vi "室外火焰对话框.vi"   [LabVIEW 2018]
types:
  T1 = enum32{"Invalid", "Standard", "Closed", "Hidden", "Minimized", "Maximized"}
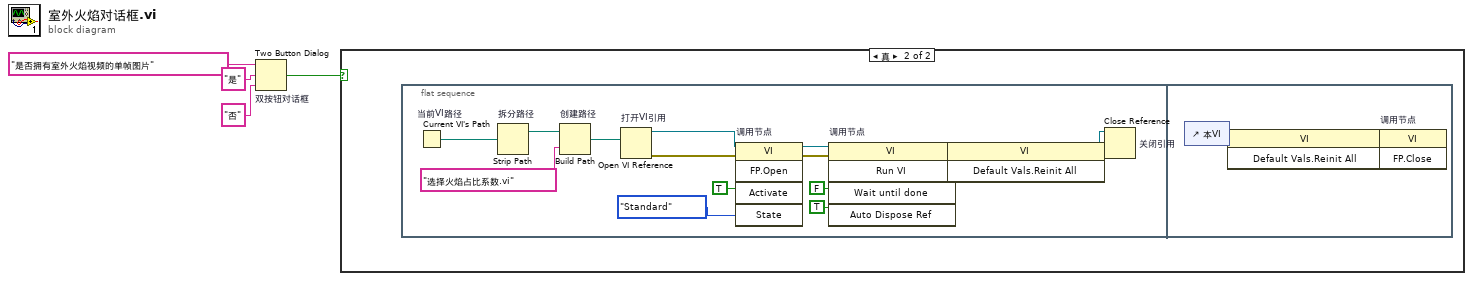
[diagram p0: block diagram]
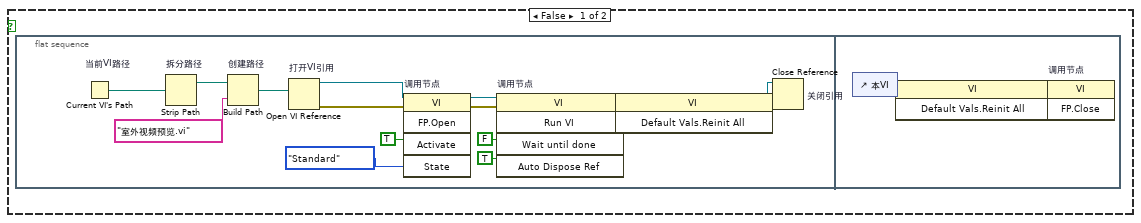
[diagram p2: hidden frame]
diagram:
  n1 = Two Button Dialog "双按钮对话框"(message="是否拥有室外火焰视频的单帧图片" ("消息"), 1:"否" ("F按钮名称（“取消”）"), 2:"是" ("T按钮名称（“确定”）")) -> (T button?=w1:bool)
  n2 = case shown="真" w1 {
    frame False {
      n3 = flat-sequence {
        frame #0 {
          n4 = Current VI's Path "当前VI路径"() -> (path=w16:path)
          n5 = Strip Path "拆分路径"(path=w16) -> (stripped path=w20:path)  [unwired: 1 out]
          n6 = Build Path "创建路径"(base path=w20, name or relative path="室外视频预览.vi" ("名称或相对路径")) -> (appended path=w17:path)
          n7 = Open VI Reference "打开VI引用"(vi path=w17) -> (vi reference=w14:refnum<vi>, error out=w13:errorcluster)  [unwired: 5 in]
          n8 = invoke on="调用节点" class="VI" method="FP.Open"(reference=w14, error in=w13, "Activate"=TRUE ("激活？"), "State"=T1."Standard" ("状态")) -> (reference out=w12:refnum<vi>, error out=w11:errorcluster)  [unwired: 1 in, 3 out]
          n9 = invoke on="调用节点" class="VI" method="Run VI"(reference=w12, error in=w11, "Wait until done"=FALSE ("结束前等待"), "Auto Dispose Ref"=TRUE ("自动销毁引用")) -> (reference out=w8:refnum<vi>, error out=w5:errorcluster)  [unwired: 1 in, 3 out]
          n10 = invoke class="VI" method="Default Vals.Reinit All"(reference=w8, error in=w5) -> (reference out=w7:refnum<vi>, error out=w6:errorcluster)  [unwired: 1 in, 1 out]
          n11 = Close Reference "关闭引用"(reference=w7, error in (no error)=w6) -> ()  [unwired: 1 out]
        }
        frame #1 {
          n12 = control-ref of="本VI"() -> (w23:refnum<vi>)
          n13 = invoke class="VI" method="Default Vals.Reinit All"(reference=w23) -> (reference out=w22:refnum<vi>, error out=w21:errorcluster)  [unwired: 2 in, 1 out]
          n14 = invoke on="调用节点" class="VI" method="FP.Close"(reference=w22, error in=w21) -> ()  [unwired: 1 in, 3 out]
        }
      }
    }
    frame True {
      n15 = flat-sequence {
        frame #0 {
          n16 = Current VI's Path "当前VI路径"() -> (path=w35:path)
          n17 = Strip Path "拆分路径"(path=w35) -> (stripped path=w39:path)  [unwired: 1 out]
          n18 = Build Path "创建路径"(base path=w39, name or relative path="选择火焰占比系数.vi" ("名称或相对路径")) -> (appended path=w36:path)
          n19 = Open VI Reference "打开VI引用"(vi path=w36) -> (vi reference=w33:refnum<vi>, error out=w32:errorcluster)  [unwired: 5 in]
          n20 = invoke on="调用节点" class="VI" method="FP.Open"(reference=w33, error in=w32, "Activate"=TRUE ("激活？"), "State"=T1."Standard" ("状态")) -> (reference out=w31:refnum<vi>, error out=w30:errorcluster)  [unwired: 1 in, 3 out]
          n21 = invoke on="调用节点" class="VI" method="Run VI"(reference=w31, error in=w30, "Wait until done"=FALSE ("结束前等待"), "Auto Dispose Ref"=TRUE ("自动销毁引用")) -> (reference out=w27:refnum<vi>, error out=w26:errorcluster)  [unwired: 1 in, 3 out]
          n22 = invoke class="VI" method="Default Vals.Reinit All"(reference=w27, error in=w26) -> (reference out=w25:refnum<vi>, error out=w24:errorcluster)  [unwired: 1 in, 1 out]
          n23 = Close Reference "关闭引用"(reference=w25, error in (no error)=w24) -> ()  [unwired: 1 out]
        }
        frame #1 {
          n24 = control-ref of="本VI"() -> (w42:refnum<vi>)
          n25 = invoke class="VI" method="Default Vals.Reinit All"(reference=w42) -> (reference out=w41:refnum<vi>, error out=w40:errorcluster)  [unwired: 2 in, 1 out]
          n26 = invoke on="调用节点" class="VI" method="FP.Close"(reference=w41, error in=w40) -> ()  [unwired: 1 in, 3 out]
        }
      }
    }
  }
